vi "Delete device.vi"(0 "Display State In":T1, 5 "Device name":string, 9 "Container State":T2, 11 "error in (no error)":errorcluster) -> (4 "Display State Out":T1, 6 "Found":bool, 15 "error out":errorcluster)   [LabVIEW 2015, in "Dynamic FP XControl.xctl"]
uses:
  Dynamic FP XControl.xctl
  <vilib>/_xctls/Container State.ctl
  Dynamic FP container.llb/Dynamic FP State.ctl
  Device/Device.lvclass
  Device/Read Name.vi
  <vilib>/_xctls/XControlSupport.lvlib
panel:
  # "Add Controls & Indicators that form the parameters of the method here. Hook them to the connector pane. Do not delete the controls & indicators that are already hooked to the connector pane.\n \nTo setup the parameters  for this method, right click on this item in the Project Tree & select \"Configure Method...\"."
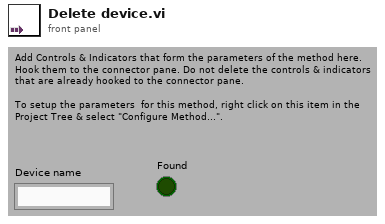
[diagram p1: front panel]
types:
  T1 = typedef "Dynamic FP XControl.xctl/Dynamic FP State.ctl" = cluster{"Complete device list":refnum<class "Device.lvclass">[], "Boolean test":bool, "Selected devices":u16[]}
  T2 = typedef "XControlSupport.lvlib/Container State.ctl" = cluster{"Indicator?":bool, "Run Mode?":bool, " Refnum":refnum<vi>}
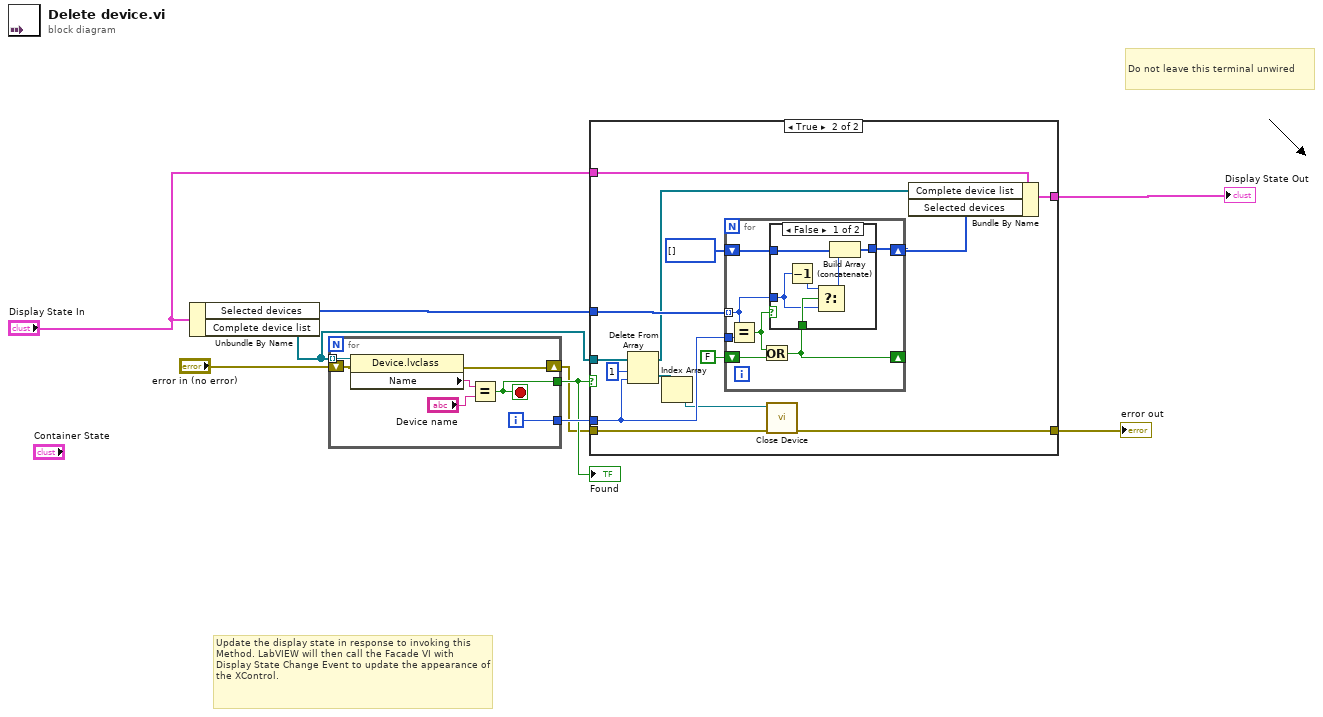
[diagram p0: block diagram]
diagram:
  # "Do not leave this terminal unwired"
  # "Update the display state in response to invoking this Method. LabVIEW will then call the Facade VI with Display State Change Event to update the appearance of the XControl."
  n1 = Unbundle By Name("Display State In") -> ("Selected devices"=w7:u16[], "Complete device list"=w8:refnum<class "Device.lvclass">[])
  n2 = for {
    tunnel: w8 -> [w16] mode=indexing
    tunnel: [w13] -> w9
    tunnel: [w12] -> w3
    shift-right: [w10] -> w2
    shift-left: "error in (no error)" -> [w11]
    i -> [w13]
    stop <- w12 stop-if-true
    n3 = property class="Device.lvclass"(reference=w16, error in=w11) -> (error out=w10:errorcluster, "Name"=w15:string)  [unwired: 1 out]
    n4 = Equal?(x=w15, y="Device name") -> (x = y?=w12:bool)
  }
  "Found" <- w3
  n5 = case shown="True" w3 {
    tunnel: w9 -> [_ w29]
    tunnel: w8 -> [_ w32]
    tunnel: w7 -> [_ w30]
    tunnel: "Display State In" -> [w18 w26]
    tunnel: [w18 w24] -> w5
    tunnel: w2 -> [w17 w20]
    tunnel: [w17 w19] -> w1
    frame False {
    }
    frame True {
      n6 = Delete From Array(array=w32, length=1, index=w29) -> (deleted portion=w22:refnum<class "Device.lvclass">[], array with subset deleted=w25:refnum<class "Device.lvclass">[])
      n7 = Index Array(array=w22) -> (element=w21:refnum<class "Device.lvclass">)  [unwired: 1 in]
      n8 = for {
        tunnel: w30 -> [w36] mode=indexing
        tunnel: w29 -> [w39]
        shift-right: [w34] -> _
        shift-left: FALSE -> [w38]
        shift-right: [w35] -> w23
        shift-left: u16[] [] -> [w33]
        n9 = Equal?(x=w36, y=w39) -> (x = y?=w37:bool)
        n10 = Or(x=w37, y=w38) -> (x .or. y?=w34:bool)
        n11 = case shown="False" w37 {
          tunnel: w36 -> [w43 _]
          tunnel: [w41 w46] -> w35
          tunnel: w34 -> [w44 _]
          tunnel: w33 -> [w40 w46]
          frame False {
            n12 = Decrement(x=w43) -> (x-1=w42:u16)
            n13 = Select(t=w42, s=w44, f=w43) -> (s? t:f=w45:u16)
            n14 = Build Array (concatenate)(w40, w45) -> (w41:u16[])
          }
          frame True {
          }
        }
      }
      n15 = call "Close Device.vi"("error in (no error)"=w20, "Device"=w21) -> ("error out"=w19:errorcluster)  [unwired: 8 in, 1 out]
      n16 = Bundle By Name(cluster=w26, "Complete device list"=w25, "Selected devices"=w23) -> (w24:T1)
    }
  }
  "Display State Out" <- w5
  "error out" <- w1
